vi "BuildPacket.vi"(1 "Data":u8[](array[numeric]), 2 "TxID":u32) -> (0 "MsgTX 2":T1)   [LabVIEW 2017]
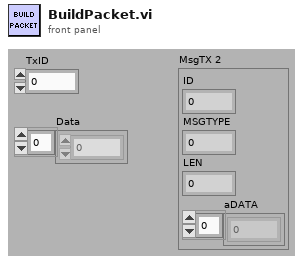
[diagram p1: front panel]
types:
  T1 = cluster{"ID":u32, "MSGTYPE":u8, "LEN":u8, "aDATA":u8[]}
  T2 = enum16{"Single SCB", "Power Rider", "Power Rider&Next10", "HATAL", "DAPH", "Indefinite", "Power Rider 12"}
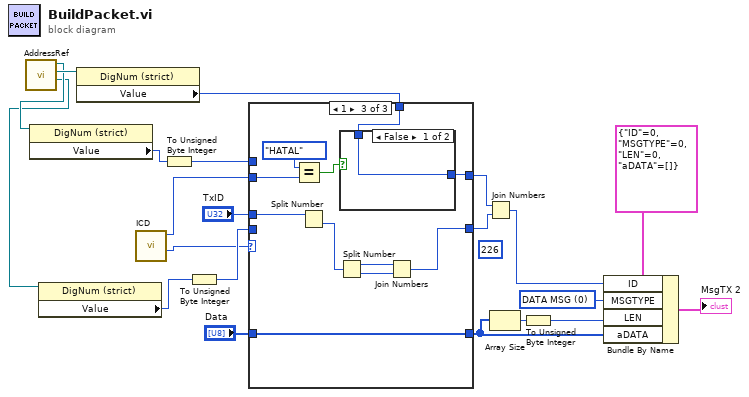
[diagram p0: block diagram]
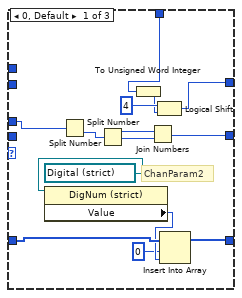
[diagram p2: hidden frame]
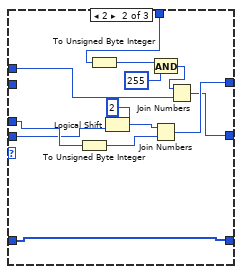
[diagram p3: hidden frame]
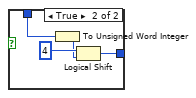
[diagram p4: hidden frame]
diagram:
  (unwired) u32 226
  w21 = u8 0 items=["STATUS"=128, "EXTENDED"=2, "RTR"=1, "DATA MSG"=0] ("MSGTYPE")
  n1 = call "AddressRef.vi"() -> ("prrty out"=w4:refnum<vi>, "add_type out"=w15:refnum<vi>, "add_dst out"=w7:refnum<vi>)  [unwired: 9 in]
  n2 = property class="DigNum (strict)"(reference=w7) -> ("Value"=w6:u16)  [unwired: 1 in, 2 out]
  n3 = property class="DigNum (strict)"(reference=w4) -> ("Value"=w3:u16)  [unwired: 1 in, 2 out]
  n4 = property class="DigNum (strict)"(reference=w15) -> ("Value"=w10:u16)  [unwired: 1 in, 2 out]
  n5 = call "ICD.vi"() -> ("UnitType"=w8:T2, "Type"=w1:u16)  [unwired: 6 in]
  n6 = To Unsigned Byte Integer(number=w6) -> (unsigned 8bit integer=w5:u8)
  n7 = To Unsigned Byte Integer(number=w3) -> (unsigned 8bit integer=w2:u8)
  n8 = case shown="1" w1 {
    tunnel: "TxID" -> [w32 w45 w59]
    tunnel: [w34 w47 w56] -> w14
    tunnel: w10 -> [w33 w46 w52]
    tunnel: [w35 w48 w53] -> w13
    tunnel: "Data" -> [w31 w42 w54]
    tunnel: [w30 w42 w54] -> w11
    tunnel: w8 -> [_ _ w49]
    tunnel: w5 -> [_ w44 _]
    tunnel: w2 -> [_ w43 _]
    frame 0, Default {
      # "ChanParam2"
      n9 = property class="DigNum (strict)"(reference=refnum<vi> refnum ("add_type out")) -> ("Value"=w24:u16)  [unwired: 1 in, 2 out]
      n10 = Split Number(x=w32) -> (lo(x)=w27:u16)  [unwired: 1 out]
      n11 = Split Number(x=w27) -> (hi(x)=w26:u8, lo(x)=w25:u8)
      n12 = To Unsigned Word Integer(number=w33) -> (unsigned 16bit integer=w28:u16)
      n13 = Join Numbers(hi=w26, lo=w25) -> ((hi.lo)=w34:u16)
      n14 = Logical Shift(y=i8 4, x=w28) -> (x << y=w35:u16)
      n15 = Insert Into Array(array=w31, index=0, new element=w24) -> (w30:u8[])
    }
    frame 2 {
      n16 = To Unsigned Byte Integer(number=w45) -> (unsigned 8bit integer=w36:u8)
      n17 = To Unsigned Byte Integer(number=w46) -> (unsigned 8bit integer=w41:u8)
      n18 = Logical Shift(y=u8 2, x=w43) -> (x << y=w37:u8)
      n19 = And(x=w41, y=u8 255) -> (x .and. y?=w39:u8)
      n20 = Join Numbers(hi=w37, lo=w36) -> ((hi.lo)=w48:u16)
      n21 = Join Numbers(hi=w39, lo=w44) -> ((hi.lo)=w47:u16)
    }
    frame 1 {
      n22 = Equal?(x=T2."HATAL" ("UnitType"), y=w49) -> (x = y?=w51:bool)
      n23 = Split Number(x=w59) -> (lo(x)=w55:u16)  [unwired: 1 out]
      n24 = Split Number(x=w55) -> (hi(x)=w57:u8, lo(x)=w58:u8)
      n25 = case shown="False" w51 {
        tunnel: [w60 w62] -> w53
        tunnel: w52 -> [w60 w61]
        frame False {
        }
        frame True {
          n26 = To Unsigned Word Integer(number=w61) -> (unsigned 16bit integer=w63:u16)
          n27 = Logical Shift(y=i8 4, x=w63) -> (x << y=w62:u16)
        }
      }
      n28 = Join Numbers(hi=w57, lo=w58) -> ((hi.lo)=w56:u16)
    }
  }
  n29 = Join Numbers(hi=w13, lo=w14) -> ((hi.lo)=w9:u32)
  n30 = Array Size(array=w11) -> (size(s)=w17:i32)
  n31 = To Unsigned Byte Integer(number=w17) -> (unsigned 8bit integer=w20:u8)
  n32 = Bundle By Name(cluster=T1 {"ID"=0, "MSGTYPE"=0, "LEN"=0, "aDATA"=[]} ("MsgTX 2"), "ID"=w9, "MSGTYPE"=w21, "LEN"=w20, "aDATA"=w11) -> (→"MsgTX 2":T1)
